vi "open_visa.vi"(8 "error in (no error)":errorcluster, 11 "VISA In":refnum<visa-resource-name>) -> (0 "error out":errorcluster, 3 "VISA Out":refnum<visa-resource-name>)   [LabVIEW 2011]
uses:
  delay_time.vi
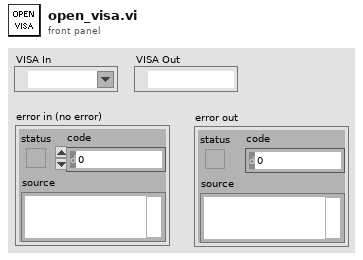
[diagram p1: front panel]
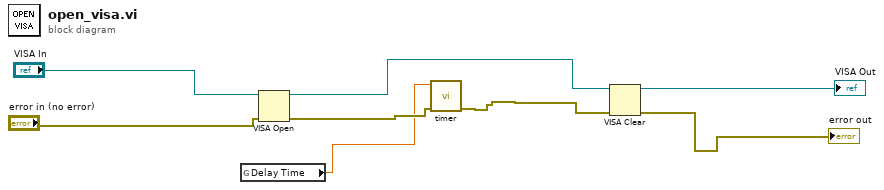
[diagram p0: block diagram]
diagram:
  n1 = global read "delay_time.vi" "Delay Time"() -> (w1:dbl)
  n2 = VISA Open(error in (no error)="error in (no error)", VISA resource name="VISA In") -> (VISA resource name=w6:refnum<visa-resource-name>, error out=w3:errorcluster)  [unwired: 3 in]
  n3 = call "timer.vi"("error in (no error)"=w3, "Delay Time"=w1) -> ("error out"=w2:errorcluster)  [unwired: 9 in]
  n4 = VISA Clear(VISA resource name=w6, error in (no error)=w2) -> (VISA resource name out=→"VISA Out":refnum<visa-resource-name>, error out=→"error out":errorcluster)
